vi "DISPLAY_QUAD.vi"(0 "VISA IN":refnum<visa-resource-name>, 5 "error in":errorcluster, 7 "Window Arrangement":string(combo)="QUAD") -> (14 "VISA Out":refnum<visa-resource-name>, 19 "error out":errorcluster)   [LabVIEW 2018, in "PNA-X.lvlib"]
doc: "DISPlay:ARRange <char> \n(Write-only) Places EXISTING measurements into pre-configured window arrangements. Overlay, \nStack(2), Split(3), and Quad(4) creates new windows. To learn more, see Arrange Existing \nMeasurements. \nParameters \n<char> Window arrangement. Choose from: \nTILE - tiles existing windows \nCASCade - overlaps existing windows \nOVERlay - all traces placed in 1 window \nSTACk - 2 windows \nSPLit - 3 windows \nQUAD - 4 windows \nExamples DISP:ARR CASC \ndisplay:arrange cascade \nQuery Syntax Not Applicable \nDefault TILE"
uses:
  PNA-X.lvlib
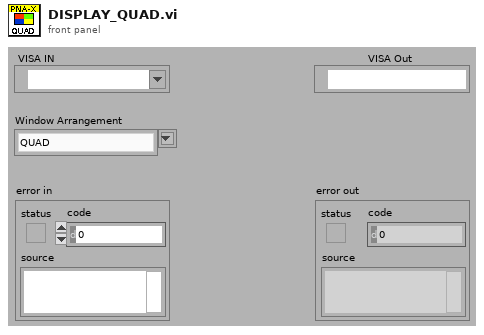
[diagram p1: front panel]
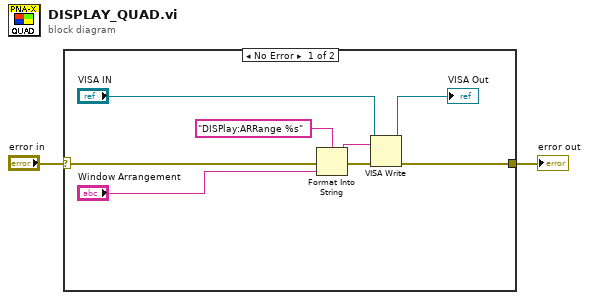
[diagram p0: block diagram]
diagram:
  n1 = case shown="No Error" "error in" {
    selector: "error in" -> [w10 w11]
    tunnel: [w5 w11] -> w1
    frame No Error {
      n2 = Format Into String(format string="DISPlay:ARRange %s" ("Cmdline"), error in=w10, "Window Arrangement") -> (resulting string=w8:string, error out=w9:errorcluster)  [unwired: 1 in]
      n3 = VISA Write(VISA resource name="VISA IN", write buffer=w8, error in (no error)=w9) -> (VISA resource name out=→"VISA Out":refnum<visa-resource-name>, error out=w5:errorcluster)  [unwired: 1 out]
    }
    frame Error {
    }
  }
  "error out" <- w1
